vi "TEST Polar Plot XControl.vi"() -> ()   [LabVIEW 2011]
doc: "Uses the Polar Graph VI to draw a polar plot in a picture indicator.\n\nNote: You must have the LabVIEW Full or Professional Development Systems to run this example.\n\nAAL 9/09"
uses:
  Polar Plot.xctl
panel:
  out "Polar Plot":cluster{"magnitude":dbl, "phase (deg)":dbl}[](xcontrol)
  in  "points":i32=180
  in  "increment":dbl=1.0 format="%0.2f"
  in  "start":dbl format="%0.2f"
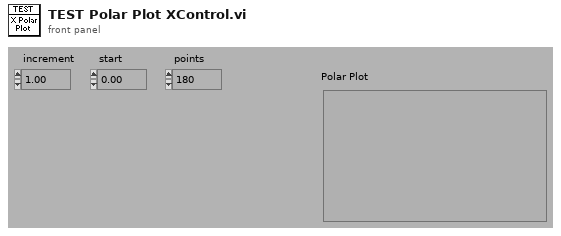
[diagram p1: front panel]
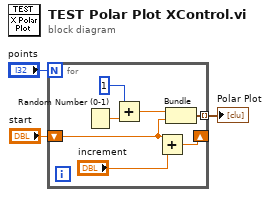
[diagram p0: block diagram]
diagram:
  n1 = for {
    N: "points" -> [_]
    tunnel: [w10] -> w1 mode=indexing
    shift-right: [w8] -> _
    shift-left: "start" -> [w7]
    n2 = Random Number (0-1)() -> (number: 0 to 1=w5:dbl)
    n3 = Add(x=1, y=w5) -> (x+y=w4:dbl)
    n4 = Add(x=w7, y="increment") -> (x+y=w8:dbl)
    n5 = Bundle(w4, "start"=w7) -> (w10:cluster{dbl, "start":dbl})  [unwired: 1 in]
  }
  "Polar Plot" <- w1
